vi "test.vi"() -> ()   [LabVIEW 2021]
panel:
  in  "stop":bool
  out "loop time":u32
  out "read buffer":string
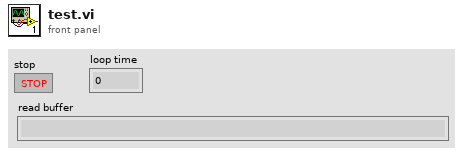
[diagram p1: front panel]
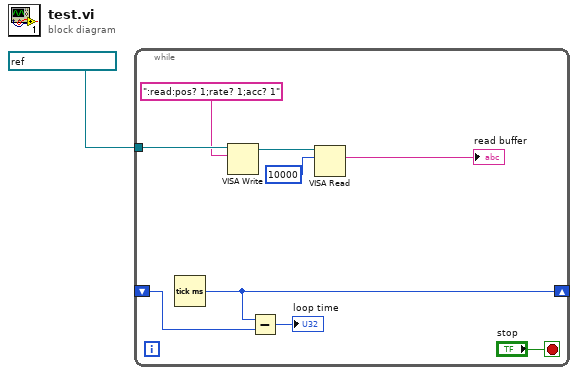
[diagram p0: block diagram]
diagram:
  n1 = while {
    tunnel: refnum<visa-resource-name> "GPIB1::1::INSTR" ("VISA resource name") -> [w10]
    shift-right: [w5] -> _
    shift-left: _ -> [w4]
    stop <- "stop" stop-if-true
    n2 = Tick Count (ms)() -> (millisecond timer value=w5:u32)
    n3 = VISA Write(VISA resource name=w10, write buffer=":read:pos? 1;rate? 1;acc? 1") -> (VISA resource name out=w8:refnum<visa-resource-name>)  [unwired: 1 in, 2 out]
    n4 = Subtract(x=w5, y=w4) -> (x-y=→"loop time":u32)
    n5 = VISA Read(VISA resource name=w8, byte count=u32 10000) -> (read buffer=→"read buffer":string)  [unwired: 1 in, 3 out]
  }
